vi "simulate.vi"(0 "angle":dbl, 1 "initialize":bool) -> (2 "standard deviation":dbl format="%0.2f", 3 "mean":dbl format="%0.2f", 4 "value":dbl)   [LabVIEW 2011]
uses:
  <vilib>/ptbypt/NI_PtbyPt.lvlib
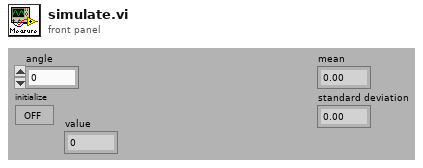
[diagram p1: front panel]
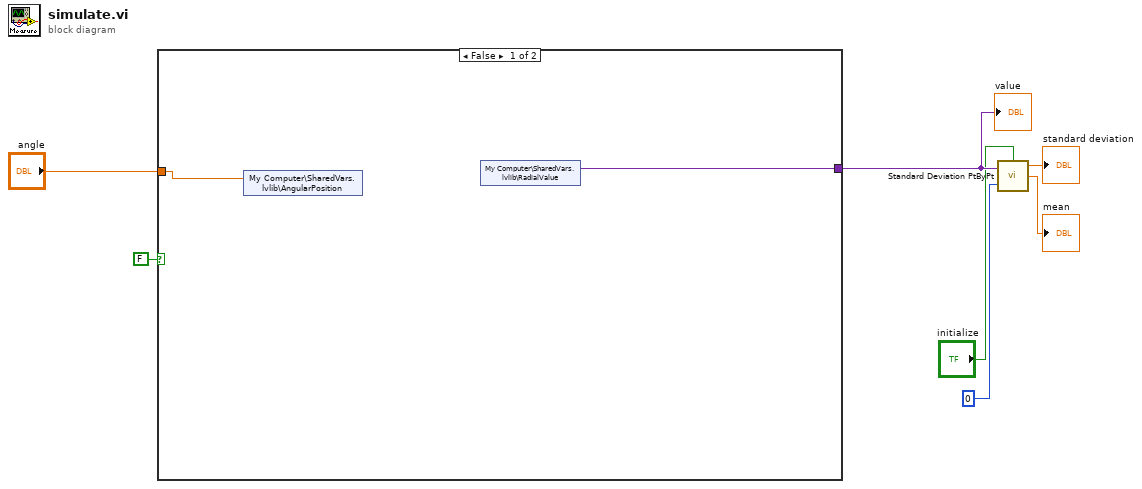
[diagram p0: block diagram]
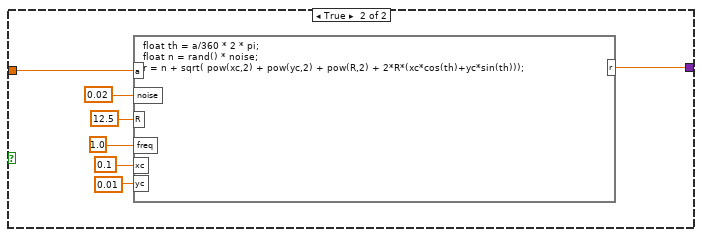
[diagram p2: hidden frame]
diagram:
  n1 = case shown="False" FALSE {
    tunnel: "angle" -> [w8 w13]
    tunnel: [w9 w12] -> w5
    frame False {
      n2 = shared-variable "My Computer\\SharedVars.lvlib\\AngularPosition"(w8) -> ()  [unwired: 1 in, 1 out]
      n3 = shared-variable "My Computer\\SharedVars.lvlib\\RadialValue"() -> (w9:variant)  [unwired: 1 in, 1 out]
    }
    frame True {
      n4 = formula code="float th = a/360 * 2 * pi;\nfloat n = rand() * noise;\nr = n + sqrt( pow(xc,2) + pow(yc,2) + pow(R,2) + 2*R*(xc*cos(th)+yc*sin(th)));"("a"=w13, "noise"=0.02 ("y"), "R"=12.5 ("y"), "freq"=1.0 ("input variable"), "xc"=0.1 ("input variable"), "yc"=0.01 ("input variable")) -> ("r"=w12:dbl)
    }
  }
  "value" <- w5
  n5 = call <vilib>:"Standard Deviation PtByPt.vi"("x"=w5, "sample length"=0, "initialize"="initialize") -> ("standard deviation"=→"standard deviation":dbl, "mean"=→"mean":dbl)  [unwired: 1 out]
